vi "rad_Deploy Image Wrapper_FB.vi"(4 "Deploy":string[](array[string]), 6 "restart after imaging (T)":bool=TRUE, 7 "Deployment Notifiers":T7, 8 "error in (no error)":errorcluster, 9 "apply primary NIC from image (F)":bool, 10 "image file path":path, 11 "Target settings in":T4={"Hostname"="", "Serial number"="", "Product name"="", "Product code"=0, "System status"="", "Credential type"=enum."None/Unlocked", "User added?"=FALSE, "Primary NIC"={"MAC address"="", "IP Address Request Mode"=2, "IP address"="", "Subnet mask"="", "Gateway"="", "DNS server"=""}, "System Credentials"={"Username"="", "Password"=""}} {"Primary NIC"."IP Address Request Mode" items=["Static"=1, "DHCP/Link-Local"=2, "Link-Local Only"=4, "DHCP Only"=8]}) -> (0 "error out":errorcluster, 2 "image file path":path, 3 "Target settings out":T4={"Hostname"="", "Serial number"="", "Product name"="", "Product code"=0, "System status"="", "Credential type"=enum."None/Unlocked", "User added?"=FALSE, "Primary NIC"={"MAC address"="", "IP Address Request Mode"=2, "IP address"="", "Subnet mask"="", "Gateway"="", "DNS server"=""}, "System Credentials"={"Username"="", "Password"=""}} {"Primary NIC"."IP Address Request Mode" items=["Static"=1, "DHCP/Link-Local"=2, "Link-Local Only"=4, "DHCP Only"=8]})   [LabVIEW 2020]
uses:
  TypeDefs/rad_Deployment Notifiers.ctl
  TypeDefs/rad_Deployment Status Data Type.ctl
  TypeDefs/rad_Deployment Progress Data Type.ctl
  support/SubVIs/Target Information.ctl
  Targets/TypeDefs/rad_Target Network Settings.ctl
  support/SubVIs/System Credentials.ctl
  <vilib>/nisyscfg/Software Set 1.2.ctl
  <vilib>/nisyscfg/Software 1.2.ctl
  <vilib>/nisyscfg/Component Type.ctl
  <vilib>/nisyscfg/Network Settings Image.ctl
  <vilib>/nisyscfg/Set System Image (Folder).vi
  <vilib>/nisyscfg/Set System Image (File).vi
  <vilib>/nisyscfg/Close (System).vi
  <vilib>/nisyscfg/nisyscfg.lvlib
  <vilib>/nisyscfg/Get Installed Set.vi
panel:
  out "Software Set":T1 {"information"."component type" items=["standard", "hidden", "system", "unknown", "startup", "image", "essential"]; "items"."component type" items=["standard", "hidden", "system", "unknown", "startup", "image", "essential"]; "add-ons"."component type" items=["standard", "hidden", "system", "unknown", "startup", "image", "essential"]}
  out "finished":bool
  in  "Stop Checking for Events":bool
  out "Progress":u8(slide) scale=0.0..100.0
  out "Status":string
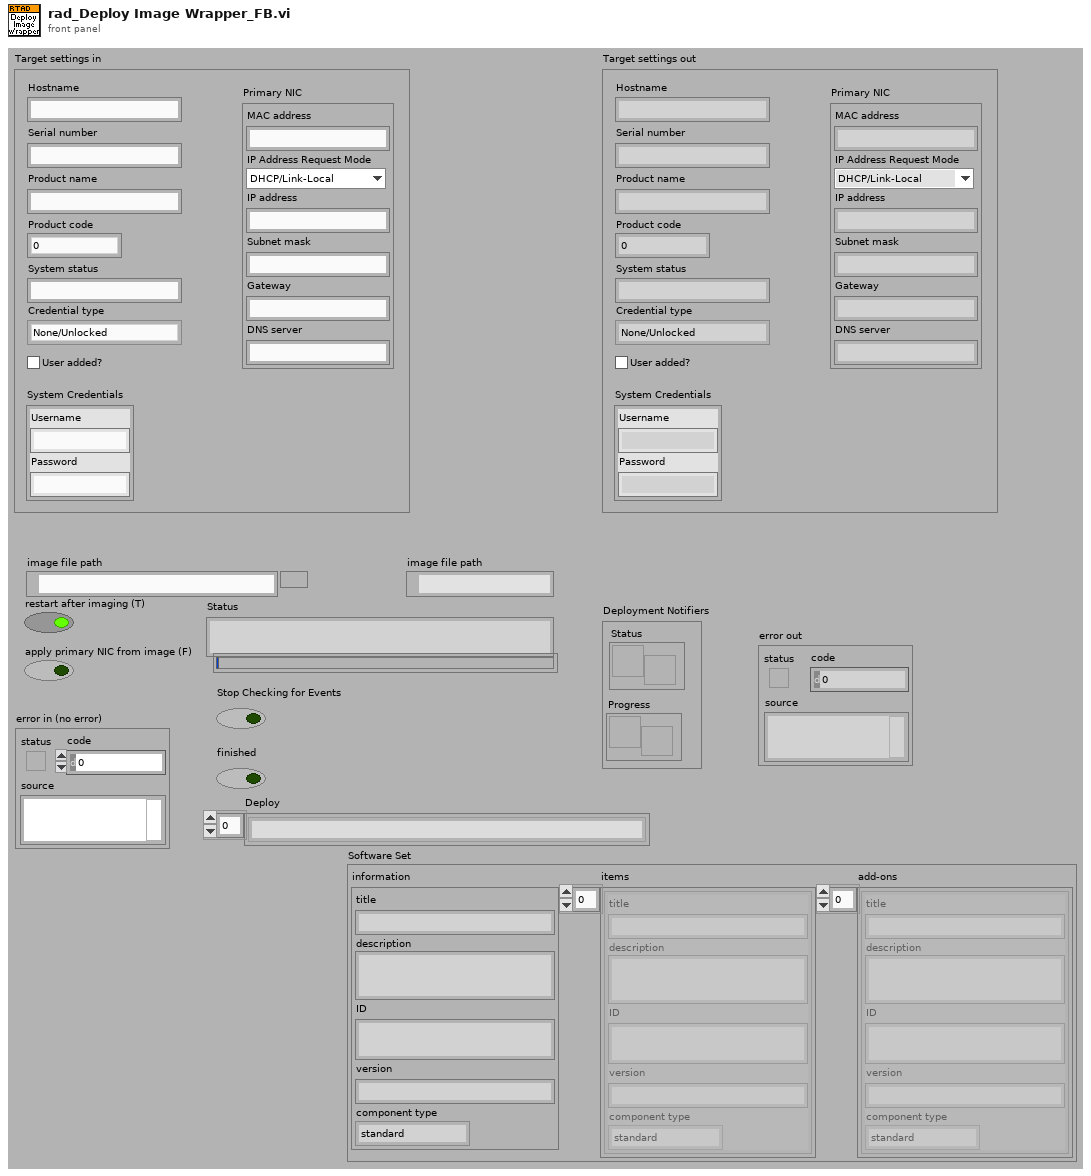
[diagram p1: front panel]
types:
  T1 = typedef "nisyscfg.lvlib/Software Set 1.2.ctl" = cluster{"information":T2, "items":T2[], "add-ons":T2[]}
  T2 = typedef "nisyscfg.lvlib/Software 1.2.ctl" = cluster{"title":string, "description":string, "ID":string, "version":string, "component type":T3}
  T3 = typedef "nisyscfg.lvlib/Component Type.ctl" = u32
  T4 = typedef "Target Information.ctl" = cluster{"Hostname":string, "Serial number":string, "Product name":string, "Product code":i32, "System status":string, "Credential type":enum16{"None/Unlocked", "FTP Password", "NIAuth Credentials"}, "User added?":bool, "Primary NIC":T5, "System Credentials":T6}
  T5 = typedef "rad_Target Network Settings.ctl" = cluster{"MAC address":string, "IP Address Request Mode":i32, "IP address":string, "Subnet mask":string, "Gateway":string, "DNS server":string}
  T6 = typedef "System Credentials.ctl" = cluster{"Username":string, "Password":string}
  T7 = typedef "rad_Deployment Notifiers.ctl" = cluster{"Status":refnum<notifier>, "Progress":refnum<notifier>}
  T8 = typedef "rad_Deployment Progress Data Type.ctl" = i8
  T9 = typedef "nisyscfg.lvlib/Network Settings Image.ctl" = u32
  T10 = enum32{"state changed", "beginning restart", "getting file", "putting file", "creating directory", "deleting file", "deleting directory", "enumerating file system", "renaming file", "current component", "operation progress", "downloading file", "unpacking file", "running install script"}
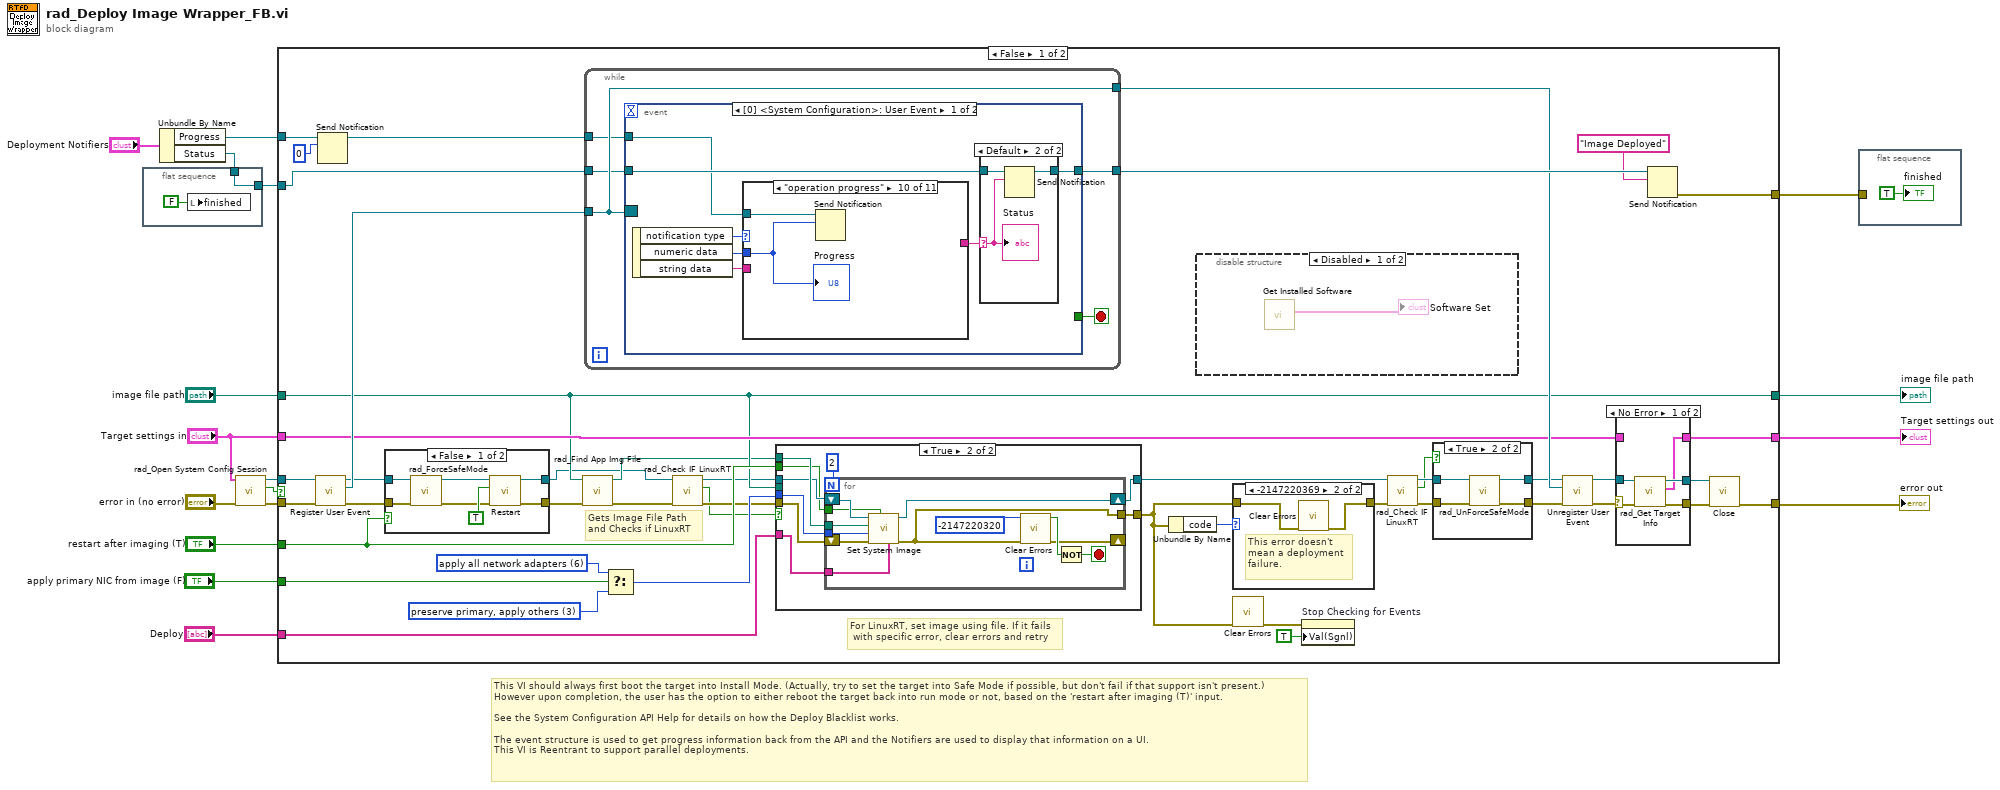
[diagram p0: block diagram]
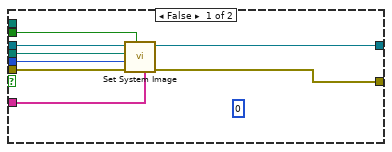
[diagram p3: hidden frame]
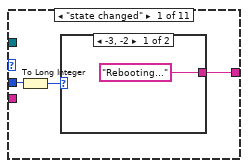
[diagram p9: hidden frame]
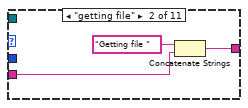
[diagram p11: hidden frame]
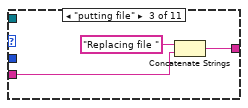
[diagram p12: hidden frame]
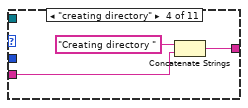
[diagram p13: hidden frame]
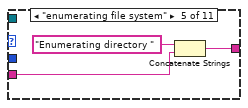
[diagram p14: hidden frame]
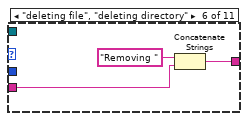
[diagram p15: hidden frame]
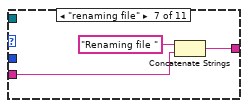
[diagram p16: hidden frame]
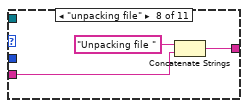
[diagram p17: hidden frame]
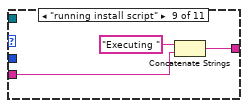
[diagram p18: hidden frame]
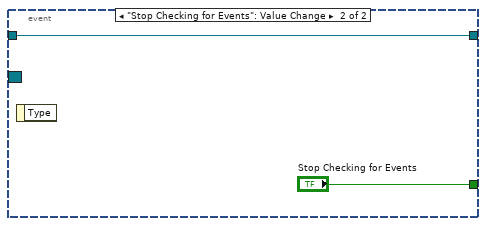
[diagram p20: hidden frame]
diagram:
  # "This VI should always first boot the target into Install Mode. (Actually, try to set the target into Safe Mode if possible, but don't fail if that support isn't present.)\nHowever upon completion, the user has the option to either reboot the target back into run mode or not, based on the 'restart after imaging (T)' input.\n\nSee the System Configuration API Help for details on how the Deploy Blacklist works.\n\nThe event structure is used to get progress information back from the API and the Notifiers are used to display that information on a UI. \nThis VI is Reentrant to support parallel deployments."
  n1 = flat-sequence {
    tunnel: [w18] -> w3
    tunnel: w2 -> [w18]
    frame #0 {
      n2 = local write "finished"(FALSE ("finished")) -> ()
    }
  }
  n3 = Unbundle By Name("Deployment Notifiers") -> ("Progress"=w11:refnum<notifier>, "Status"=w2:refnum<notifier>)
  n4 = call "rad_Open System Config Session.vi"("error in (no error)"="error in (no error)", "Target settings"="Target settings in") -> ("error out"=w7:errorcluster, "Cancelled"=w6:bool, "Session out"=w8:refnum<k21>)  [unwired: 6 in, 1 out]
  n5 = case shown="False" w6 {
    tunnel: [w64 w171] -> w17
    tunnel: "image file path" -> [w32 w170]
    tunnel: "restart after imaging (T)" -> [w48 _]
    tunnel: w8 -> [w63 _]
    tunnel: w7 -> [w62 w171]
    tunnel: [w58 _] -> w14
    tunnel: "apply primary NIC from image (F)" -> [w20 _]
    tunnel: w11 -> [w54 _]
    tunnel: [w32 w170] -> w16
    tunnel: "Deploy" -> [w34 _]
    tunnel: "Target settings in" -> [w35 w169]
    tunnel: [w45 w169] -> w4
    tunnel: w3 -> [w41 _]
    frame False {
      w57 = T9 6 items=["reset primary, disable others", "preserve primary, disable others", "preserve all network adapters", "preserve primary, apply others", "apply primary, disable others", "apply primary, preserve others", "apply all network adapters"] ("network settings (apply all adapters)")
      w56 = T9 3 items=["reset primary, disable others", "preserve primary, disable others", "preserve all network adapters", "preserve primary, apply others", "apply primary, disable others", "apply primary, preserve others", "apply all network adapters"] ("network settings (apply all adapters)")
      # "Gets Image File Path\nand Checks if LinuxRT"
      # "For LinuxRT, set image using file. If it fails\n with specific error, clear errors and retry"
      n6 = call <vilib>:"Register User Event.vi"("error in (no error)"=w62, "Session in"=w63) -> ("error out"=w49:errorcluster, "Event Registration out"=w61:refnum<event-registration>, "Session out"=w50:refnum<k21>)  [unwired: 7 in]
      n7 = Send Notification(notification=T8 0, notifier=w54) -> (notifier out=w53:refnum<notifier>)  [unwired: 1 in, 1 out]
      n8 = case shown="False" w48 {
        tunnel: w50 -> [w115 w117]
        tunnel: w49 -> [w110 w116]
        tunnel: [w113 w117] -> w29
        tunnel: [w112 w116] -> w33
        frame False {
          n9 = call "rad_ForceSafeMode.vi"("error in (no error)"=w110, "Target in"=w115) -> ("error out"=w109:errorcluster, "Target out"=w111:refnum<k21>)  [unwired: 8 in]
          n10 = call <vilib>:"Restart.vi"("error in (no error)"=w109, "Install Mode (F)"=TRUE ("install mode (F)"), "Session in"=w111) -> ("error out"=w112:errorcluster, "Session out"=w113:refnum<k21>)  [unwired: 6 in, 1 out]
        }
        frame True {
        }
      }
      n11 = call "rad_Find App Img File.vi"("Error In"=w33, "Temp Image Path"=w32) -> ("Error Out"=w30:errorcluster, "LVAppImg Path"=w31:path)  [unwired: 8 in]
      n12 = while {
        tunnel: w61 -> [w125]
        tunnel: [w125] -> w44
        tunnel: w41 -> [w123]
        tunnel: [w122] -> w60
        tunnel: w53 -> [w121]
        stop <- w124 stop-if-true
        n13 = event shown="[0] <System Configuration>: User Event" {
          selector: w125 -> [_ _]
          dyn-events: _ -> [_ _]
          timeout: _ -> [_ _]
          tunnel: [_ "Stop Checking for Events"] -> w124
          tunnel: w123 -> [w128 w167]
          tunnel: [w127 w167] -> w122
          tunnel: w121 -> [w126 _]
          event User Event {
            n14 = event-data() -> ("notification type"=w132:T10, "numeric data"=w130:u32, "string data"=w131:string)  [unwired: 1 in]
            n15 = case shown="\"operation progress\"" w132 {
              tunnel: [w137 w141 w144 w147 w150 w153 w156 w159 w162 _ _] -> w129
              tunnel: w131 -> [_ w142 w145 w148 w151 w154 w157 w160 w163 _ _]
              tunnel: w130 -> [w139 _ _ _ _ _ _ _ _ w166 _]
              tunnel: w126 -> [_ _ _ _ _ _ _ _ _ w165 _]
              frame "state changed" {
                n16 = To Long Integer(number=w139) -> (32bit integer=w138:i32)
                n17 = case shown="-3, -2" w138 {
                  tunnel: ["Rebooting..." _] -> w137
                  frame -3, -2 {
                  }
                  frame Default {
                  }
                }
              }
              frame "getting file" {
                n18 = Concatenate Strings("Getting file " ("Status"), w142) -> (w141:string)
              }
              frame "putting file" {
                n19 = Concatenate Strings("Replacing file " ("Status"), w145) -> (w144:string)
              }
              frame "creating directory" {
                n20 = Concatenate Strings("Creating directory " ("Status"), w148) -> (w147:string)
              }
              frame "enumerating file system" {
                n21 = Concatenate Strings("Enumerating directory " ("Status"), w151) -> (w150:string)
              }
              frame "deleting file", "deleting directory" {
                n22 = Concatenate Strings("Removing " ("Status"), w154) -> (w153:string)
              }
              frame "renaming file" {
                n23 = Concatenate Strings("Renaming file " ("Status"), w157) -> (w156:string)
              }
              frame "unpacking file" {
                n24 = Concatenate Strings("Unpacking file " ("Status"), w160) -> (w159:string)
              }
              frame "running install script" {
                n25 = Concatenate Strings("Executing " ("Status"), w163) -> (w162:string)
              }
              frame "operation progress" {
                n26 = Send Notification(notification=w166, notifier=w165) -> ()  [unwired: 1 in, 2 out]
                "Progress" <- w166
              }
              frame Default {
              }
            }
            n27 = case shown="Default" w129 {
              selector: w129 -> [_ w135]
              tunnel: w128 -> [w133 w136]
              tunnel: [w133 w134] -> w127
              frame "" {
              }
              frame Default {
                n28 = Send Notification(notification=w135, notifier=w136) -> (notifier out=w134:refnum<notifier>)  [unwired: 1 in, 1 out]
                "Status" <- w135
              }
            }
          }
          event "Stop Checking for Events": Value Change {
            n29 = event-data() -> ()  [unwired: 1 in, 1 out]
          }
        }
      }
      n30 = Select(t=w57, s=w20, f=w56) -> (s? t:f=w55:T9)
      n31 = call "rad_Check IF LinuxRT.vi"("Error In"=w30, "System Session In"=w29) -> ("Error Out"=w27:errorcluster, "Target is LinuxRT?"=w26:bool, "System Session Out"=w28:refnum<k21>)  [unwired: 5 in, 2 out]
      n32 = case shown="True" w26 {
        tunnel: w55 -> [w69 w79]
        tunnel: w32 -> [w70 _]
        tunnel: w28 -> [w71 w81]
        tunnel: w27 -> [w68 w78]
        tunnel: w48 -> [w72 w80]
        tunnel: [w66 w75] -> w39
        tunnel: [w73 w74] -> w23
        tunnel: w34 -> [w67 w76]
        tunnel: w31 -> [_ w82]
        frame False {
          (unwired) 0
          n33 = call-poly <vilib>:"Set System Image.vi"("File and Directory Blacklist"=w67, "Restart Automatically (T)"=w72, "error in (no error)"=w68, "Network Settings (preserve primary adapter, apply others)"=w69, "Source Folder"=w70, "Session in"=w71) -> ("error out"=w66:errorcluster, "Session out"=w73:refnum<k21>)  [unwired: 4 in]
        }
        frame True {
          n34 = for {
            N: 2 -> [_]
            tunnel: w82 -> [w94]
            tunnel: w80 -> [w92]
            tunnel: w79 -> [w91]
            tunnel: w76 -> [w89]
            tunnel: [w84] -> w75
            shift-right: [w86] -> _
            shift-left: w78 -> [w90]
            shift-right: [w85] -> w74
            shift-left: w81 -> [w93]
            stop <- w88 stop-if-true
            n35 = call-poly <vilib>:"Set System Image.vi"("File and Directory Blacklist"=w89, "Restart Automatically (T)"=w92, "error in (no error)"=w90, "Network Settings (preserve primary adapter, apply others)"=w91, "Source File"=w94, "Session in"=w93) -> ("error out"=w84:errorcluster, "Session out"=w85:refnum<k21>)  [unwired: 4 in]
            n36 = call <vilib>:"Clear Errors.vi"("error in (no error)"=w84, "specific error code to clear (0: all)"=-2147220320) -> ("error out"=w86:errorcluster, "specific error cleared?"=w87:bool)  [unwired: 4 in]
            n37 = Not(x=w87) -> (.not. x?=w88:bool)
          }
        }
      }
      n38 = Unbundle By Name(w39) -> ("code"=w51:i32)
      n39 = disable-structure shown="Disabled" {
        frame Disabled {
          n40 = call-poly <vilib>:"Get Installed Software.vi"() -> ("Software Set"=→"Software Set":T1)  [unwired: 9 in, 2 out]
        }
        frame Enabled {
        }
      }
      n41 = case shown="-2147220369" w51 {
        tunnel: w39 -> [w118 w120]
        tunnel: [w118 w119] -> w25
        frame Default {
        }
        frame -2147220369 {
          # "This error doesn't\nmean a deployment\nfailure."
          n42 = call <vilib>:"Clear Errors.vi"("error in (no error)"=w120) -> ("error out"=w119:errorcluster)  [unwired: 5 in, 1 out]
        }
      }
      n43 = call <vilib>:"Clear Errors.vi"("error in (no error)"=w39) -> ("error out"=w38:errorcluster)  [unwired: 5 in, 1 out]
      n44 = property on="Stop Checking for Events" class="Bool (strict)"(error in=w38, "Val(Sgnl)"=TRUE ("Stop Checking for Events")) -> ()  [unwired: 1 in, 2 out]
      n45 = call "rad_Check IF LinuxRT.vi"("Error In"=w25, "System Session In"=w23) -> ("Error Out"=w24:errorcluster, "Target is LinuxRT?"=w21:bool, "System Session Out"=w22:refnum<k21>)  [unwired: 5 in, 2 out]
      n46 = case shown="True" w21 {
        tunnel: w22 -> [w96 w100]
        tunnel: w24 -> [w95 w99]
        tunnel: [w95 w97] -> w37
        tunnel: [w96 w98] -> w36
        frame False {
        }
        frame True {
          n47 = call "rad_UnForceSafeMode.vi"("error in (no error)"=w99, "Target in"=w100) -> ("error out"=w97:errorcluster, "Target out"=w98:refnum<k21>)  [unwired: 8 in]
        }
      }
      n48 = call <vilib>:"Unregister User Event.vi"("error in (no error)"=w37, "Event Registration in"=w44, "Session in"=w36) -> ("error out"=w43:errorcluster, "Session out"=w42:refnum<k21>)  [unwired: 7 in]
      n49 = case shown="No Error" w43 {
        selector: w43 -> [w104 w108]
        tunnel: [w102 w108] -> w47
        tunnel: w42 -> [w105 w107]
        tunnel: [w103 w107] -> w46
        tunnel: [w101 w106] -> w45
        tunnel: w35 -> [_ w106]
        frame No Error {
          n50 = call "rad_Get Target Info.vi"("error in (no error)"=w104, "System Session in"=w105) -> ("error out"=w102:errorcluster, "Target settings"=w101:T4, "System Session out"=w103:refnum<k21>)  [unwired: 7 in]
        }
        frame Error {
        }
      }
      n51 = Send Notification(notification="Image Deployed", notifier=w60) -> (error out=w58:errorcluster)  [unwired: 1 in, 1 out]
      n52 = call-poly <vilib>:"Close.vi"("error in (no error)"=w47, "Session in"=w46) -> ("error out"=w64:errorcluster)  [unwired: 9 in]
    }
    frame True {
    }
  }
  "error out" <- w17
  "image file path" <- w16
  "Target settings out" <- w4
  n53 = flat-sequence {
    tunnel: w14 -> [_]
    frame #0 {
      "finished" <- TRUE ("finished")
    }
  }
